vi "toggle_controls.vi"(8 "error in":errorcluster, 9 "setup ID":i32, 10 "vars general in":T1[](array[typedef]) {"stim ramp" min=1}, 11 "control cluster in":T4) -> (0 "error out":errorcluster, 1 "setup ID":i32, 2 "vars general out":T1[](array[typedef]) {"stim ramp" min=1}, 3 "control cluster out":T4)   [LabVIEW 2016]
uses:
  Type Definitions/control_references.ctl
  Type Definitions/vars_settings.ctl
  Type Definitions/stim_type.ctl
  Type Definitions/backlight_type.ctl
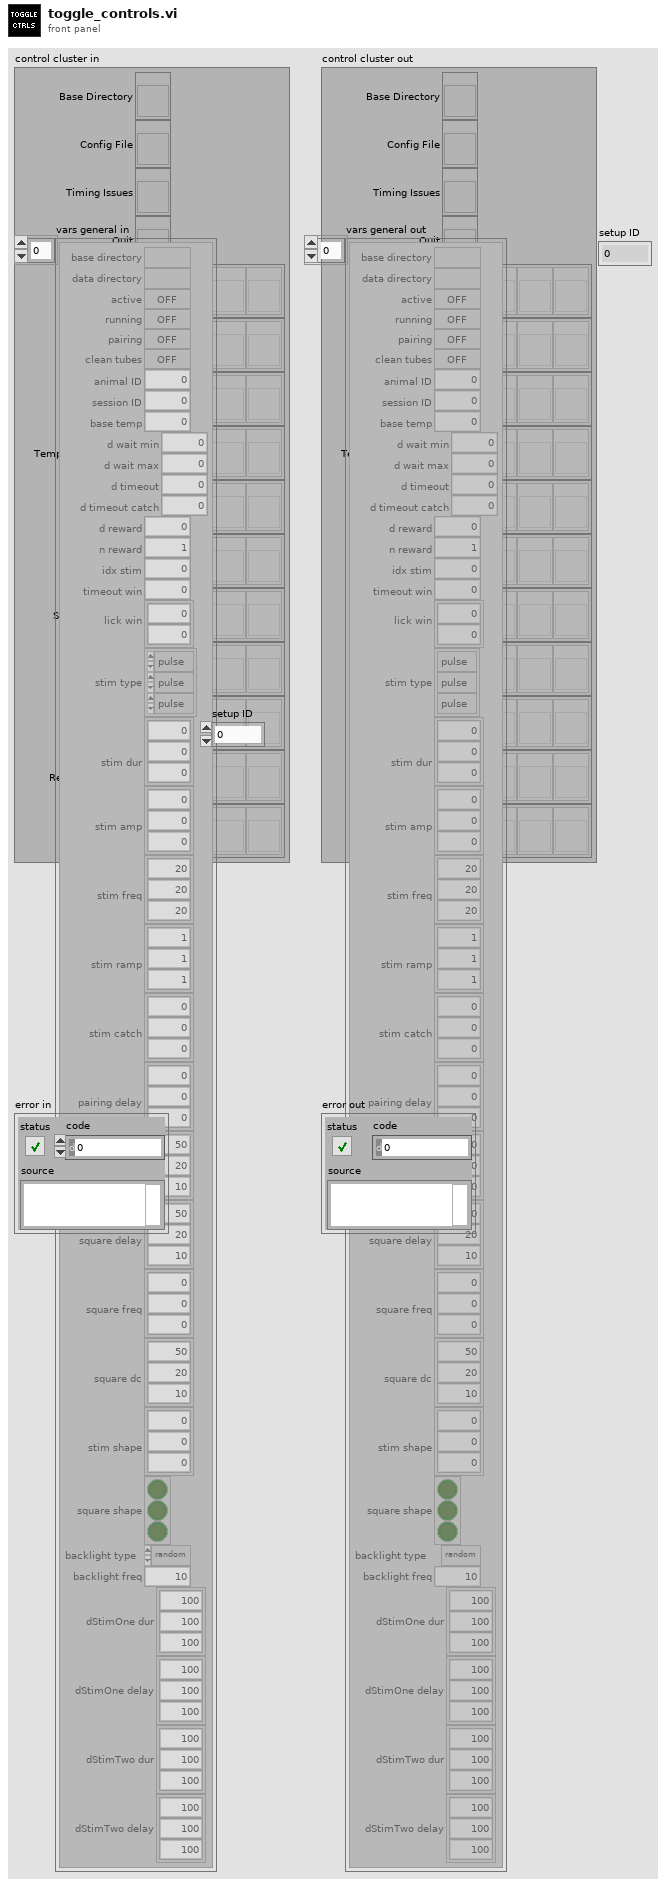
[diagram p1: front panel]
types:
  T1 = typedef "vars_settings.ctl" = cluster{"base directory":path, "data directory":path, "active":bool, "running":bool, "pairing":bool, "clean tubes":bool, "animal ID":u16, "session ID":u16, "base temp":dbl, "d wait min":u16, "d wait max":u16, "d timeout":u16, "d timeout catch":u16, "d reward":u16, "n reward":u16, "idx stim":u16, "timeout win":u16, "lick win":i32[], "stim type":T2[], "stim dur":u16[], "stim amp":dbl[], "stim freq":u16[], "stim ramp":u16[], "stim catch":u8[], "pairing delay":i16[], "square dur":u16[], "square delay":i16[], "square freq":u8[], "square dc":u8[], "stim shape":dbl[][], "square shape":bool[][], "backlight type":T3, "backlight freq":u16, "dStimOne dur":u16[], "dStimOne delay":i16[], "dStimTwo dur":u16[], "dStimTwo delay":i16[]}
  T2 = typedef "stim_type.ctl" = enum16{"pulse", "vibration", "square", "sine"}
  T3 = typedef "backlight_type.ctl" = enum16{"none", "random", "regular"}
  T4 = typedef "control_references.ctl" = cluster{"Base Directory":refnum<vi>, "Config File":refnum<vi>, "Timing Issues":refnum<vi>, "Quit":refnum<vi>, "Animal ID":refnum<vi>[], "Session ID":refnum<vi>[], "Active":refnum<vi>[], "Temperature Charts":refnum<vi>[], "Lick Charts":refnum<vi>[], "Bool Displays":refnum<vi>[], "Stimulus Timing":refnum<vi>[], "Stimulus Stats":refnum<vi>[], "Catch Stats":refnum<vi>[], "Recording Status":refnum<vi>[], "Pairing":refnum<vi>[]}
  T5 = enum8{"Enabled", "Disabled", "Disabled and Grayed Out"}
  T6 = enum8{"Enabled", "Disabled", "Disabled and Grayed Out"}[]
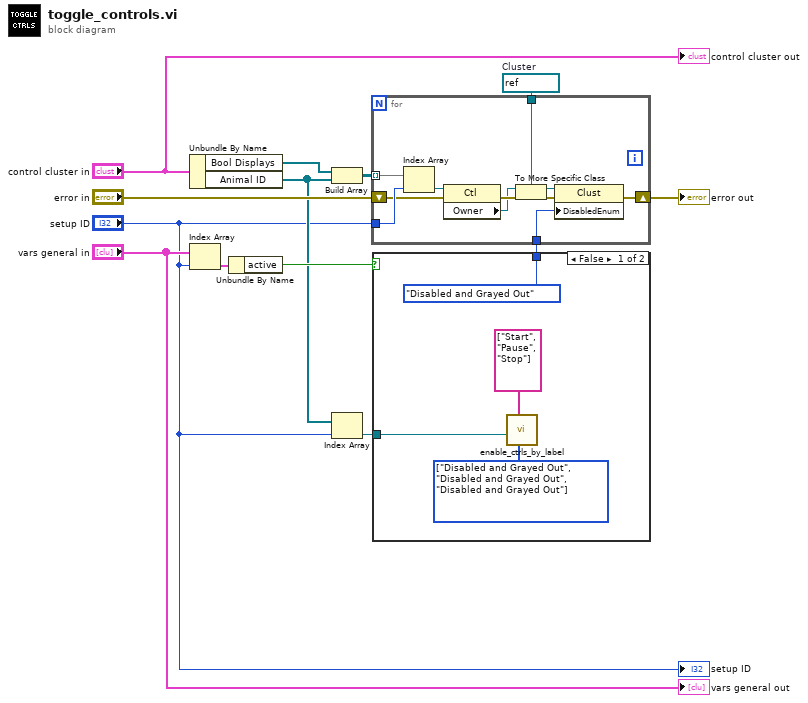
[diagram p0: block diagram]
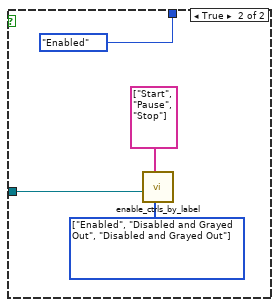
[diagram p2: hidden frame]
diagram:
  w10 = refnum<vi> refnum  # Cluster
  n1 = Unbundle By Name("control cluster in") -> ("Bool Displays"=w12:refnum<vi>[], "Animal ID"=w2:refnum<vi>[])
  n2 = Index Array(array="vars general in", index="setup ID") -> (element=w8:T1)
  n3 = Unbundle By Name(w8) -> ("active"=w6:bool)
  n4 = Build Array(w12, w2) -> (w11:refnum<vi>[][])
  n5 = Index Array(array=w2, index="setup ID") -> (element=w3:refnum<vi>)
  n6 = case shown="False" w6 {
    tunnel: [T5."Disabled and Grayed Out" ("Disabled") T5."Enabled" ("Disabled")] -> w5
    tunnel: w3 -> [w16 w20]
    frame False {
      w15 = T6 [enum."Disabled and Grayed Out", enum."Disabled and Grayed Out", enum."Disabled and Grayed Out"] items=["Enabled", "Disabled", "Disabled and Grayed Out"] ("State")
      n7 = call "enable_ctrls_by_label.vi"("States"=w15, "Names"=string[] ["Start", "Pause", "Stop"], "Refnum in"=w16) -> ()  [unwired: 7 in, 2 out]
    }
    frame True {
      w19 = T6 [enum."Enabled", enum."Disabled and Grayed Out", enum."Disabled and Grayed Out"] items=["Enabled", "Disabled", "Disabled and Grayed Out"] ("State")
      n8 = call "enable_ctrls_by_label.vi"("States"=w19, "Names"=string[] ["Start", "Pause", "Stop"], "Refnum in"=w20) -> ()  [unwired: 7 in, 2 out]
    }
  }
  n9 = for {
    tunnel: w11 -> [w32] mode=indexing
    tunnel: "setup ID" -> [w31]
    tunnel: w10 -> [w28]
    shift-right: [w24] -> w4
    shift-left: "error in" -> [w25]
    tunnel: w5 -> [w22]
    n10 = Index Array(array=w32, index=w31) -> (element=w30:refnum<vi>)
    n11 = property class="Ctl"(reference=w30, error in=w25) -> (error out=w29:errorcluster, "Owner"=w23:refnum<vi>)  [unwired: 1 out]
    n12 = To More Specific Class(target class=w28, reference=w23, error in=w29) -> (specific class reference=w27:refnum<vi>, error out=w26:errorcluster)
    n13 = property class="Clust"(reference=w27, error in=w26, "DisabledEnum"=w22) -> (error out=w24:errorcluster)  [unwired: 1 out]
  }
  "error out" <- w4
  "control cluster out" <- "control cluster in"
  "vars general out" <- "vars general in"
  "setup ID" <- "setup ID"
